vi "SID_oscillator.vi"(4 "reset phase":bool=TRUE, 5 "sampling info":cluster{"Fs":dbl, "#s":i32}={"Fs"=44100.0, "#s"=50}, 6 "MSB in":bool, 7 "Reg":T1 {"Duty" format="%0.2f"; "ADSR"."R" format="%0.2f"; "ADSR"."S" format="%0.2f"; "ADSR"."D" format="%0.2f"; "ADSR"."A" format="%0.2f"; "freq" format="%0.2f"}) -> (2 "MSB out":bool, 3 "wave":dbl[](array[numeric]))   [LabVIEW 2018]
uses:
  SID_voice_reg.ctl
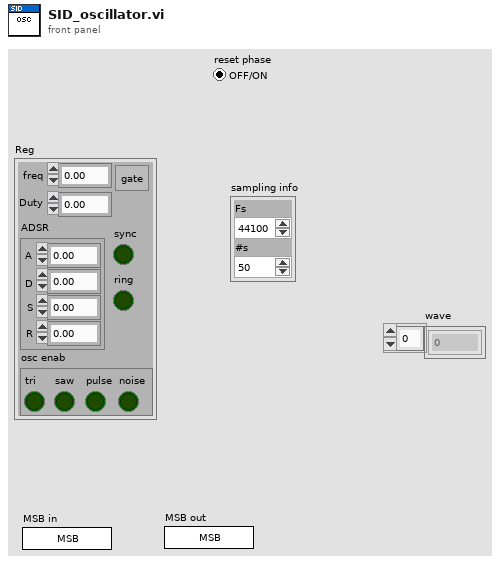
[diagram p1: front panel]
types:
  T1 = typedef "SID_voice_reg.ctl" = cluster{"freq":dbl, "gate":bool, "ADSR":cluster{"A":dbl, "D":dbl, "S":dbl, "R":dbl}, "Duty":dbl, "osc enab":cluster{"tri":bool, "saw":bool, "pulse":bool, "noise":bool}, "sync":bool, "ring":bool}
  T2 = cluster{"tri":bool, "saw":bool, "pulse":bool, "noise":bool}
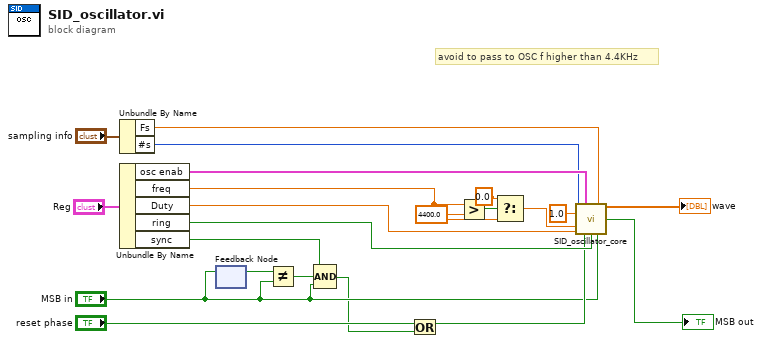
[diagram p0: block diagram]
diagram:
  # "avoid to pass to OSC f higher than 4.4KHz"
  n1 = Unbundle By Name("sampling info") -> ("Fs"=w18:dbl, "#s"=w19:i32)
  n2 = Unbundle By Name("Reg") -> ("osc enab"=w20:T2, "freq"=w10:dbl, "Duty"=w14:dbl, "ring"=w8:bool, "sync"=w2:bool)
  n3 = feedback-in #1("MSB in") -> ()
  n4 = feedback #1() -> (w5:bool)  [unwired: 1 in]
  n5 = Not Equal?(x=w5, y="MSB in") -> (x != y?=w4:bool)
  n6 = Compound Arithmetic op=AND(w2, w4, "MSB in") -> (w1:bool)
  n7 = Or(x="reset phase", y=w1) -> (x .or. y?=w6:bool)
  n8 = Greater?(x=w10, y=4400.0) -> (0:w12:bool)
  n9 = Select(t=0.0 ("amplitude"), s=w12, f=w10) -> (s? t:f=w9:dbl)
  n10 = call "SID_oscillator_core.vi"("samples"=w19, "wave enab"=w20, "Fs"=w18, "amplitude"=1.0, "freq"=w9, "pulse width"=w14, "reset"=w6, "use ext OSC"=w8, "MSB in"="MSB in") -> ("wave"=→"wave":dbl[], "MSB out"=→"MSB out":bool)  [unwired: 4 in, 1 out]
